vi "Global Variables.vi"() -> ()   [LabVIEW 2014]
panel:
  out "LifterVictor_Value":dbl
  out "Rotation":dbl
  out "Y_Axis":dbl
  out "X_Axis":dbl
  out "LifterDownButton":bool
  out "LifterUpButton":bool
  out "LowerLimitSwitch_Lifter":bool
  out "UpperLimitSwitch_Lifter":bool
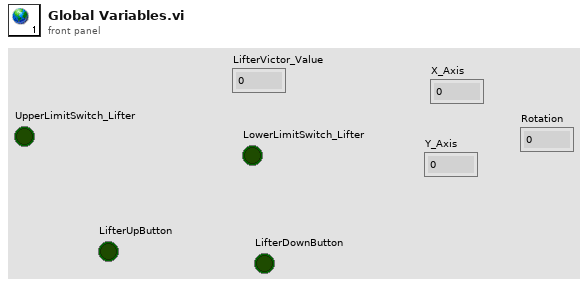
[diagram p1: front panel]
diagram:
